vi "Handle Error.vi"(8 "error in (no error)":errorcluster, 11 "IModel in":refnum<class "IModel.lvclass">) -> (0 "error out":errorcluster, 2 "stop actor?":bool=TRUE, 3 "IModel out":refnum<class "IModel.lvclass">)   [LabVIEW 2018, in "MVA Framework.lvlib" / "IModel.lvlib" / "IModel.lvclass"]
doc: "(<B>Filename</B>: Actor Framework.lvlib:Actor.lvclass:Handle Error.vi)\n\nDefines how the actor handles an error that occurred while processing a message. By default, this method does nothing except stop the actor."
uses:
  IModel.lvclass
  <vilib>/ActorFramework/Actor/Actor.lvclass
  <vilib>/ActorFramework/Stop Msg/Stop Msg.lvclass
  IObserver/IObserver/IObserver.lvclass
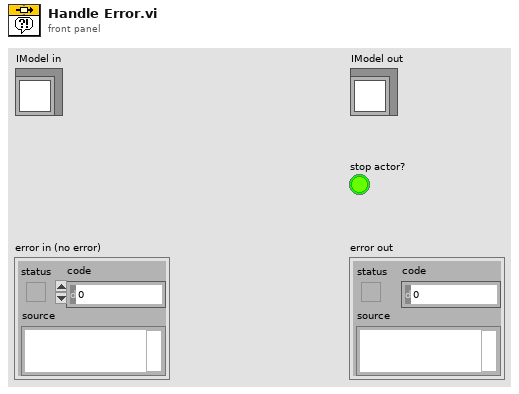
[diagram p1: front panel]
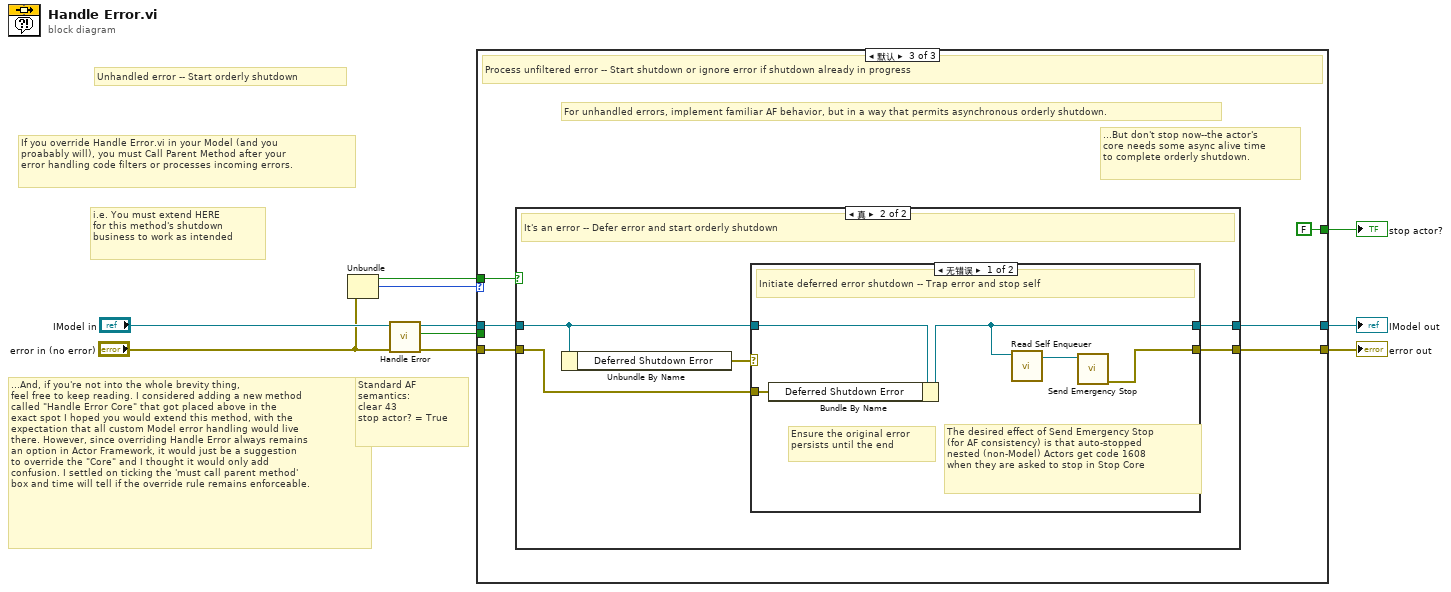
[diagram p0: block diagram]
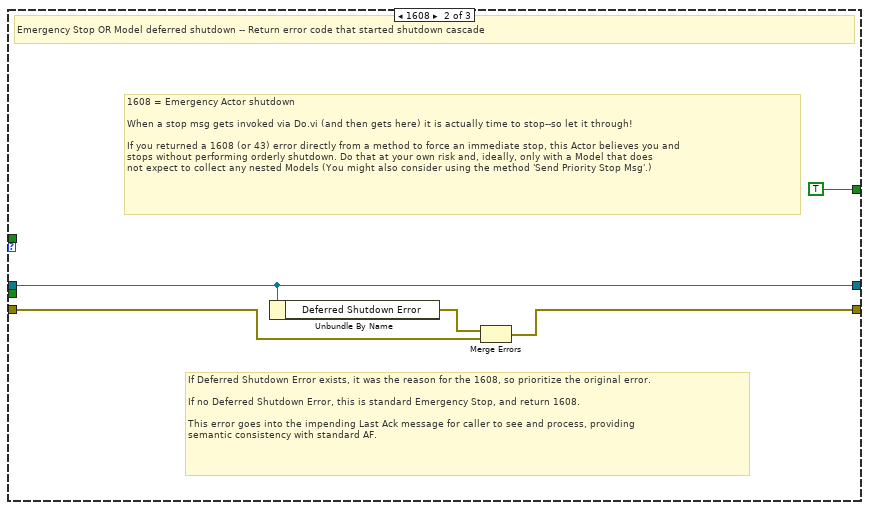
[diagram p3: hidden frame]
diagram:
  # "Standard AF\nsemantics:\nclear 43\nstop actor? = True"
  # "Unhandled error -- Start orderly shutdown"
  # "...And, if you're not into the whole brevity thing,\nfeel free to keep reading. I considered adding a new method\ncalled \"Handle Error Core\" that got placed above in the\nexact spot I hoped you would extend this method, with the\nexpectation that all custom Model error handling would live\nthere. However, since overriding Handle Error always remains\nan option in Actor Framework, it would just be a suggestion\nto override the \"Core\" and I thought it would only add\nconfusion. I settled on ticking the 'must call parent method'\nbox and time will tell if the override rule remains enforceable."
  # "i.e. You must extend HERE\nfor this method's shutdown\nbusiness to work as intended"
  # "If you override Handle Error.vi in your Model (and you\nproabably will), you must Call Parent Method after your\nerror handling code filters or processes incoming errors."
  n1 = Unbundle("error in (no error)") -> ("status"=w3:bool, "code"=w8:i32)  [unwired: 1 out]
  n2 = call-parent "Handle Error.vi"("error in (no error)"="error in (no error)", "IObserver in"="IModel in") -> ("error out"=w5:errorcluster, "stop actor?"=w4:bool, "IObserver out"=w6:refnum<class "IModel.lvclass">)  [unwired: 7 in]
  n3 = case shown="默认" w8 {
    tunnel: w5 -> [w13 w15 w19]
    tunnel: w6 -> [w12 w18 w22]
    tunnel: [w12 w18 w20] -> w10
    tunnel: [w13 w14 w24] -> w9
    tunnel: [w11 TRUE ("stop actor?") FALSE ("stop actor?")] -> w7
    tunnel: w4 -> [w11 _ _]
    tunnel: w3 -> [_ _ w21]
    frame 43 {
      # "43 = Normal Actor shutdown\n\nWhen a stop msg gets invoked via Do.vi (and then gets here) it is actually time to stop--so let it through!\n\nIf you returned a 43 (or 1608) error directly from a method to force an immediate stop, this Actor believes you and\nstops without performing orderly shutdown. Do that at your own risk and, ideally, only with a Model that does\nnot expect to collect any nested Models (You might also consider using the method 'Send Priority Stop Msg'.)"
      # "Handle normal Actor shutdown code"
    }
    frame 1608 {
      # "1608 = Emergency Actor shutdown\n\nWhen a stop msg gets invoked via Do.vi (and then gets here) it is actually time to stop--so let it through!\n\nIf you returned a 1608 (or 43) error directly from a method to force an immediate stop, this Actor believes you and\nstops without performing orderly shutdown. Do that at your own risk and, ideally, only with a Model that does\nnot expect to collect any nested Models (You might also consider using the method 'Send Priority Stop Msg'.)"
      # "If Deferred Shutdown Error exists, it was the reason for the 1608, so prioritize the original error.\n\nIf no Deferred Shutdown Error, this is standard Emergency Stop, and return 1608.\n\nThis error goes into the impending Last Ack message for caller to see and process, providing\nsemantic consistency with standard AF."
      # "Emergency Stop OR Model deferred shutdown -- Return error code that started shutdown cascade"
      n4 = Unbundle By Name(w18) -> ("Deferred Shutdown Error"=w16:errorcluster)
      n5 = Merge Errors(w16, w15) -> (w14:errorcluster)
    }
    frame Default {
      # "For unhandled errors, implement familiar AF behavior, but in a way that permits asynchronous orderly shutdown."
      # "...But don't stop now--the actor's\ncore needs some async alive time\nto complete orderly shutdown."
      # "Process unfiltered error -- Start shutdown or ignore error if shutdown already in progress"
      n6 = case shown="真" w21 {
        tunnel: [_ w30] -> w24
        tunnel: w22 -> [w25 w29]
        tunnel: [w25 w28] -> w20
        tunnel: w19 -> [_ w26]
        frame False {
          # "Error was cleared or it's just a warning (Unlike Actors, Models ignore warnings)"
        }
        frame True {
          # "It's an error -- Defer error and start orderly shutdown"
          n7 = Unbundle By Name(w29) -> ("Deferred Shutdown Error"=w27:errorcluster)
          n8 = case shown="无错误" w27 {
            tunnel: [w34 _] -> w30
            tunnel: w29 -> [w33 w36]
            tunnel: [w32 w36] -> w28
            tunnel: w26 -> [w31 _]
            frame No Error {
              # "Ensure the original error\npersists until the end"
              # "The desired effect of Send Emergency Stop\n(for AF consistency) is that auto-stopped\nnested (non-Model) Actors get code 1608\nwhen they are asked to stop in Stop Core"
              # "Initiate deferred error shutdown -- Trap error and stop self"
              n9 = Bundle By Name(cluster=w33, "Deferred Shutdown Error"=w31) -> (w32:refnum<class "IModel.lvclass">)
              n10 = call <vilib>:"Read Self Enqueuer.vi"("Actor"=w32) -> ("Self Enqueuer"=w35:refnum<class "Message Enqueuer.lvclass">)  [unwired: 10 in]
              n11 = call <vilib>:"Send Emergency Stop.vi"("Message Enqueuer"=w35) -> ("error out"=w34:errorcluster)  [unwired: 10 in]
            }
            frame Error {
              # "Error-based shutdown already in progress--\ndo not update code, do not resend e-stop,\ndo not collect one million dollars."
              # "Deferred error shutdown already in progress"
            }
          }
        }
      }
    }
  }
  "IModel out" <- w10
  "error out" <- w9
  "stop actor?" <- w7
